vi "Write Fast FPGA Telem to TDMS.vi"   [LabVIEW 2015]
uses:
  FPGA Telem for Fast Logging.ctl
  Global Data.vi
types:
  T1 = enum16{"open", "open or create", "create or replace", "create", "open (read-only)"}
  T2 = cluster{"read mode":enum16{"polling", "blocking"}, "write mode":enum16{"polling", "blocking"}}
  T3 = typedef "FPGA Telem for Fast Logging.ctl" = cluster{"Time Stamp":timestamp, "tRequestMCControl":dbl, "rAverageThrottle":dbl, "rTPS2":fxp<+/-,31,22>, "rTPS1":fxp<+/-,31,22>, "rThrottle":fxp<+/-,33,22>, "aSteerWheel":fxp<+/-,31,13>, "pBrakeR":fxp<+,26,13>, "pBrakeF":fxp<+,26,13>, "ILowCurrent":fxp<+/-,24,15>, "IHighCurrent":fxp<+/-,24,15>, "nWheelFL":fxp<+/-,32,16>, "nWheelFR":fxp<+/-,32,16>, "nWheelRL":fxp<+/-,32,16>, "nWheelRR":fxp<+/-,32,16>, "gXiPhone":dbl, "gYiPhone":dbl, "gZiPhone":dbl, "nYawXiPhone":dbl, "nYawYiPhone":dbl, "nYawZiPhone":dbl, "vWheelRR":fxp<+/-,32,18>, "vWheelRL":fxp<+/-,32,18>, "vWheelFR":fxp<+/-,32,18>, "vWheelFL":fxp<+/-,32,18>, "vWheelLowest":fxp<+/-,32,18>, "vWheelHighest":fxp<+/-,32,18>, "vAxleF":fxp<+/-,33,19>, "vCar":fxp<+/-,33,19>, "sLap":fxp<+,32,12>, "rSlipRL":fxp<+/-,12,1>, "rSlipRR":fxp<+/-,12,1>, "rSlipFL":fxp<+/-,12,1>, "rSlipFR":fxp<+/-,12,1>, "MPowerLimiterCorrection":dbl}
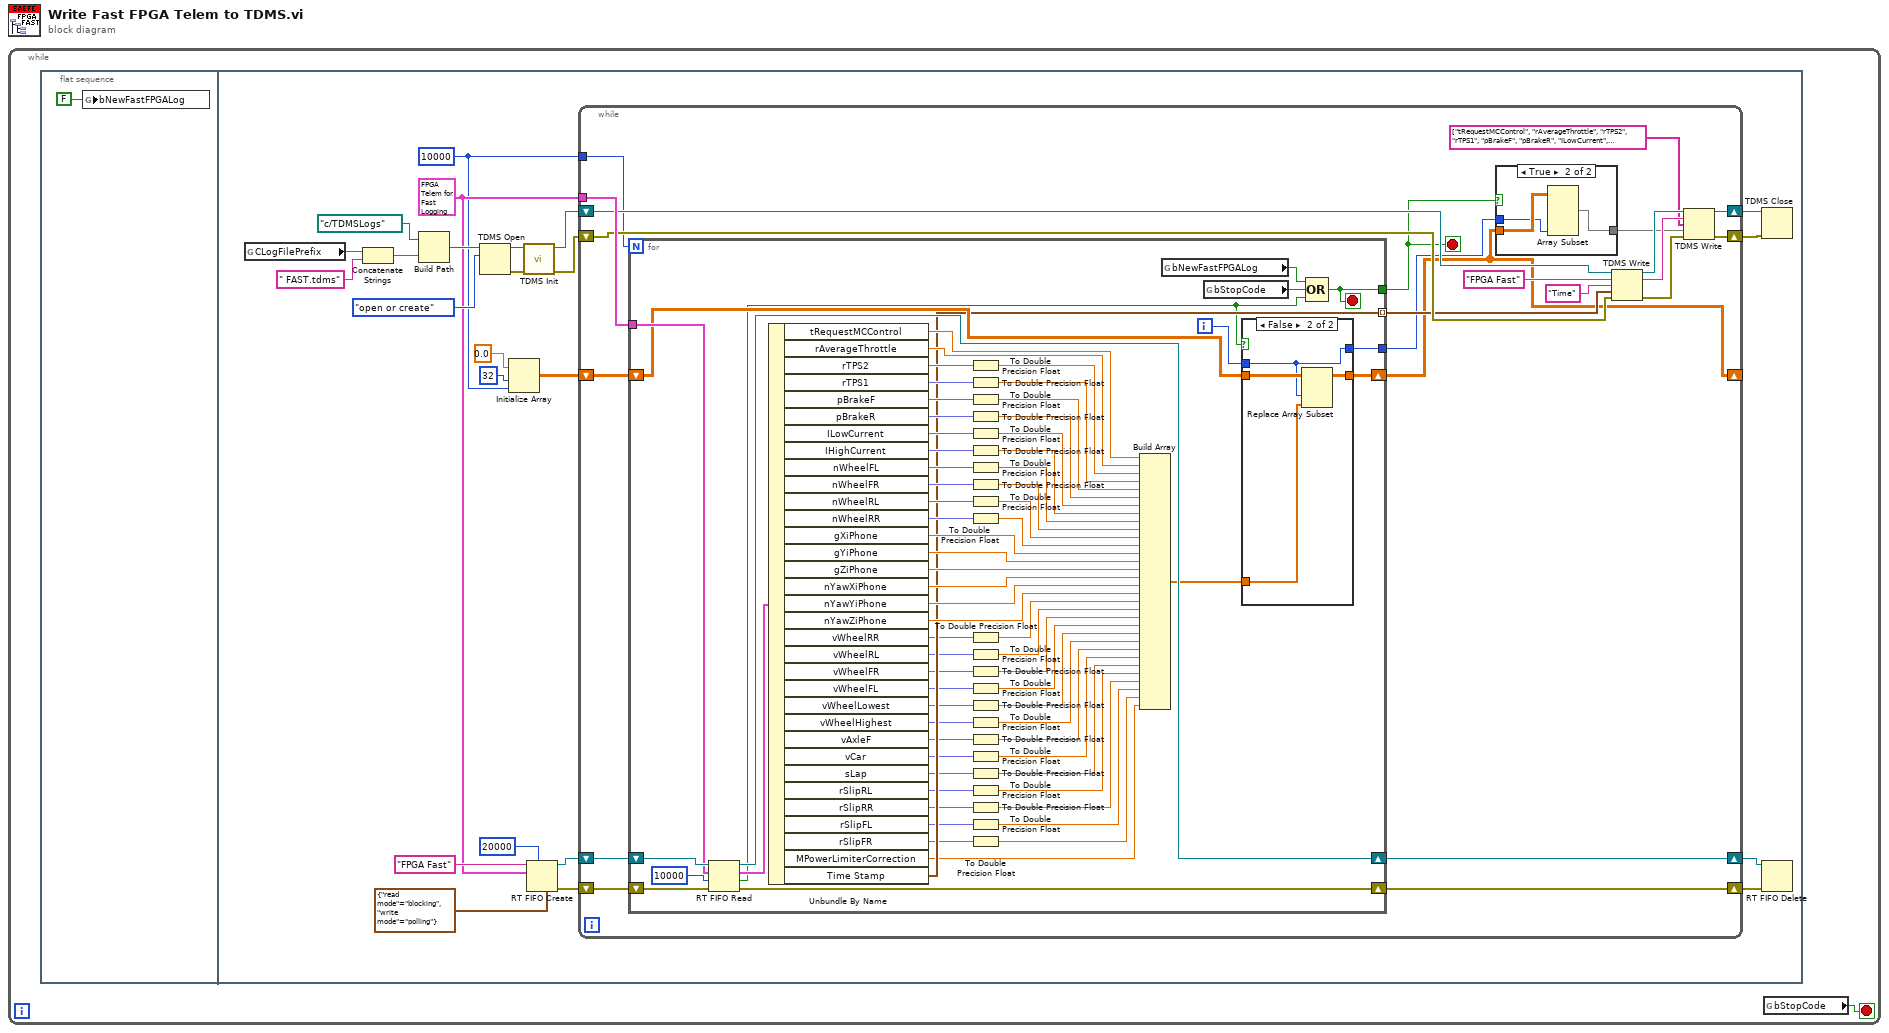
[diagram p0: block diagram]
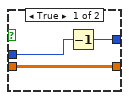
[diagram p3: hidden frame]
diagram:
  n1 = while {
    stop <- w1 stop-if-true
    n2 = flat-sequence {
      frame #0 {
        n3 = global write "Global Data.vi" "bNewFastFPGALog"(FALSE ("New F_FPGA TDMS")) -> ()
      }
      frame #1 {
        w3 = 10000 ("dimension size")
        w10 = T3 {"Time Stamp"=timestamp(0 s since 1904-01-01), "tRequestMCControl"=0.0, "rAverageThrottle"=0.0, "rTPS2"=0.421875, "rTPS1"=0.69921875, "rThrottle"=0.0, "aSteerWheel"=0.0078125, "pBrakeR"=186.34033203125, "pBrakeF"=185.44775390625, "ILowCurrent"=0.48046875, "IHighCurrent"=0.482421875, "nWheelFL"=0.0, "nWheelFR"=0.0, "nWheelRL"=0.0, "nWheelRR"=0.0, "gXiPhone"=0.0, "gYiPhone"=0.0, "gZiPhone"=0.0, "nYawXiPhone"=0.0, "nYawYiPhone"=0.0, "nYawZiPhone"=0.0, "vWheelRR"=0.0, "vWheelRL"=0.0, "vWheelFR"=0.0, "vWheelFL"=0.0, "vWheelLowest"=0.0, "vWheelHighest"=0.0, "vAxleF"=0.0, "vCar"=0.0, "sLap"=0.0, "rSlipRL"=0.0, "rSlipRR"=0.0, "rSlipFL"=0.0, "rSlipFR"=0.0, "MPowerLimiterCorrection"=0.0} ("FPGA Fast Telem")
        n4 = global read "Global Data.vi" "CLogFilePrefix"() -> (w6:string)
        n5 = Concatenate Strings(w6, " FAST.tdms" ("string")) -> (w4:string)
        n6 = Build Path(base path=path "c:/TDMSLogs", name or relative path=w4) -> (appended path=w21:path)
        n7 = TDMS Open(10:T1."open or create" ("operation (0:open)"), 11:w21) -> (0:w15:errorcluster, 3:w16:refnum<k34>)  [unwired: 5 in]
        n8 = Initialize Array(0.0 ("element"), 32 ("dimension size"), w3) -> (w7:dbl[][])
        n9 = call "TDMS Init.vi"("error in (no error)"=w15, "tdms file"=w16) -> ("error out"=w13:errorcluster, "tdms file out"=w14:refnum<k34>)  [unwired: 8 in]
        n10 = RT FIFO Create(0:"FPGA Fast" ("name (unnamed)"), 1:w10, 4:u32 20000 ("size (10)"), 7:T2 {"read mode"=enum."blocking", "write mode"=enum."polling"} ("r/w modes (polling,polling)")) -> (8:w23:refnum<k33>, 11:w22:errorcluster)  [unwired: 4 in, 1 out]
        n11 = while {
          tunnel: w10 -> [w46]
          shift-right: [w45] -> w11
          shift-left: w23 -> [w48]
          shift-right: [w44] -> w12
          shift-left: w22 -> [w47]
          shift-right: [w34] -> w18
          shift-left: w14 -> [w43]
          shift-right: [w33] -> w17
          shift-left: w13 -> [w42]
          shift-right: [w30] -> _
          shift-left: w7 -> [w32]
          tunnel: w3 -> [w28]
          stop <- w27 stop-if-true
          n12 = for {
            N: w28 -> [_]
            tunnel: w46 -> [w122]
            shift-right: [w120] -> w45
            shift-left: w48 -> [w124]
            shift-right: [w119] -> w44
            shift-left: w47 -> [w123]
            tunnel: [w83] -> w41 mode=indexing
            shift-right: [w103] -> w30
            shift-left: w32 -> [w104]
            tunnel: [w53] -> w29
            tunnel: [w55] -> w27
            i -> [w102]
            stop <- w55 stop-if-true
            n13 = RT FIFO Read(0:w124, 1:w122, 2:10000 ("timeout in ms (0)"), 3:w123) -> (8:w120:refnum<k33>, 9:w118:T3, 10:w54:bool, 11:w119:errorcluster)  [unwired: 1 out]
            n14 = Unbundle By Name(w118) -> ("tRequestMCControl"=w98:dbl, "rAverageThrottle"=w99:dbl, "rTPS2"=w117:fxp<+/-,31,22>, "rTPS1"=w116:fxp<+/-,31,22>, "pBrakeF"=w115:fxp<+,26,13>, "pBrakeR"=w114:fxp<+,26,13>, "ILowCurrent"=w113:fxp<+/-,24,15>, "IHighCurrent"=w112:fxp<+/-,24,15>, "nWheelFL"=w97:fxp<+/-,32,16>, "nWheelFR"=w96:fxp<+/-,32,16>, "nWheelRL"=w95:fxp<+/-,32,16>, "nWheelRR"=w94:fxp<+/-,32,16>, "gXiPhone"=w89:dbl, "gYiPhone"=w88:dbl, "gZiPhone"=w87:dbl, "nYawXiPhone"=w86:dbl, "nYawYiPhone"=w85:dbl, "nYawZiPhone"=w84:dbl, "vWheelRR"=w82:fxp<+/-,32,18>, "vWheelRL"=w81:fxp<+/-,32,18>, "vWheelFR"=w80:fxp<+/-,32,18>, "vWheelFL"=w79:fxp<+/-,32,18>, "vWheelLowest"=w78:fxp<+/-,32,18>, "vWheelHighest"=w77:fxp<+/-,32,18>, "vAxleF"=w76:fxp<+/-,33,19>, "vCar"=w75:fxp<+/-,33,19>, "sLap"=w74:fxp<+,32,12>, "rSlipRL"=w73:fxp<+/-,12,1>, "rSlipRR"=w72:fxp<+/-,12,1>, "rSlipFL"=w71:fxp<+/-,12,1>, "rSlipFR"=w70:fxp<+/-,12,1>, "MPowerLimiterCorrection"=w56:dbl, "Time Stamp"=w83:timestamp)
            n15 = To Double Precision Float(number=w117) -> (double precision float=w111:dbl)
            n16 = To Double Precision Float(number=w116) -> (double precision float=w110:dbl)
            n17 = To Double Precision Float(number=w115) -> (double precision float=w109:dbl)
            n18 = To Double Precision Float(number=w114) -> (double precision float=w108:dbl)
            n19 = To Double Precision Float(number=w113) -> (double precision float=w107:dbl)
            n20 = To Double Precision Float(number=w112) -> (double precision float=w106:dbl)
            n21 = To Double Precision Float(number=w97) -> (double precision float=w93:dbl)
            n22 = To Double Precision Float(number=w96) -> (double precision float=w92:dbl)
            n23 = To Double Precision Float(number=w95) -> (double precision float=w91:dbl)
            n24 = To Double Precision Float(number=w94) -> (double precision float=w90:dbl)
            n25 = To Double Precision Float(number=w82) -> (double precision float=w69:dbl)
            n26 = To Double Precision Float(number=w81) -> (double precision float=w68:dbl)
            n27 = To Double Precision Float(number=w80) -> (double precision float=w67:dbl)
            n28 = To Double Precision Float(number=w79) -> (double precision float=w66:dbl)
            n29 = To Double Precision Float(number=w78) -> (double precision float=w65:dbl)
            n30 = To Double Precision Float(number=w77) -> (double precision float=w64:dbl)
            n31 = To Double Precision Float(number=w76) -> (double precision float=w63:dbl)
            n32 = To Double Precision Float(number=w75) -> (double precision float=w62:dbl)
            n33 = To Double Precision Float(number=w74) -> (double precision float=w61:dbl)
            n34 = To Double Precision Float(number=w73) -> (double precision float=w60:dbl)
            n35 = To Double Precision Float(number=w72) -> (double precision float=w59:dbl)
            n36 = To Double Precision Float(number=w71) -> (double precision float=w58:dbl)
            n37 = To Double Precision Float(number=w70) -> (double precision float=w57:dbl)
            n38 = Build Array(w98, w99, w111, w110, w109, w108, w107, w106, w93, w92, w91, w90, w89, w88, w87, w86, w85, w84, w69, w68, w67, w66, w65, w64, w63, w62, w61, w60, w59, w58, w57, w56) -> (w105:dbl[])
            n39 = global read "Global Data.vi" "bNewFastFPGALog"() -> (w101:bool)
            n40 = global read "Global Data.vi" "bStopCode"() -> (w100:bool)
            n41 = case shown="False" w54 {
              tunnel: w105 -> [_ w131]
              tunnel: w104 -> [w127 w130]
              tunnel: [w127 w129] -> w103
              tunnel: w102 -> [w126 w128]
              tunnel: [w125 w128] -> w53
              frame True {
                n42 = Decrement(x=w126) -> (x-1=w125:i32)
              }
              frame False {
                n43 = Replace Array Subset(array=w130, new element=w131, index (col)=w128) -> (w129:dbl[][])  [unwired: 1 in]
              }
            }
            n44 = Compound Arithmetic op=OR(w101, w100, w54) -> (w55:bool)
          }
          n45 = case shown="True" w27 {
            tunnel: w30 -> [w49 w52]
            tunnel: [w49 w50] -> w31
            tunnel: w29 -> [_ w51]
            frame False {
            }
            frame True {
              n46 = Array Subset(array=w52, length (col)=w51) -> (w50:dbl[][])  [unwired: 3 in]
            }
          }
          n47 = TDMS Write(0:w43, 5:"FPGA Fast" ("group name in (Untitled)"), 7:"Time", 9:w41, 11:w42) -> (4:w38:refnum<k34>, 6:w36:string, 15:w37:errorcluster)  [unwired: 1 in, 1 out]
          n48 = TDMS Write(0:w38, 5:w36, 7:string[] ["tRequestMCControl", "rAverageThrottle", "rTPS2", "rTPS1", "pBrakeF", "pBrakeR", "ILowCurrent", "IHighCurrent", "nWheelFL", "nWheelFR", "nWheelRL", "nWheelRR", "gXiPhone", "gYiPhone", "gZiPhone", "nYawXiPhone", "nYawYiPhone", "nYawZiPhone", "vWheelRR", "vWheelRL", "vWheelFR", "vWheelFL", "vWheelLowest", "vWheelHighest", "vAxleF", "vCar", "sLap", "rSlipRL", "rSlipRR", "rSlipFL", "rSlipFR", "MPowerLimiterCorrection"] ("channel name(s) in (Untitled)"), 9:w31, 11:w37) -> (4:w34:refnum<k34>, 15:w33:errorcluster)  [unwired: 1 in, 2 out]
        }
        n49 = TDMS Close(8:w17, 11:w18) -> ()  [unwired: 2 out]
        n50 = RT FIFO Delete(0:w11, 3:w12) -> ()  [unwired: 1 in, 1 out]
      }
    }
    n51 = global read "Global Data.vi" "bStopCode"() -> (w1:bool)
  }
